vi "Set Socket.vi"(8 "error in (no error)":errorcluster, 11 "Channel Pub in":refnum<class "Channel Pub.lvclass">) -> (0 "error out":errorcluster, 3 "Channel Pub out":refnum<class "Channel Pub.lvclass">)   [LabVIEW 2018, in "Channel Pub.lvclass"]
uses:
  Channel Pub.lvclass
  Communication Channel/Communication Channel Folder/Communication Channel.lvclass
  Socket2/Socket2/Socket2.lvclass
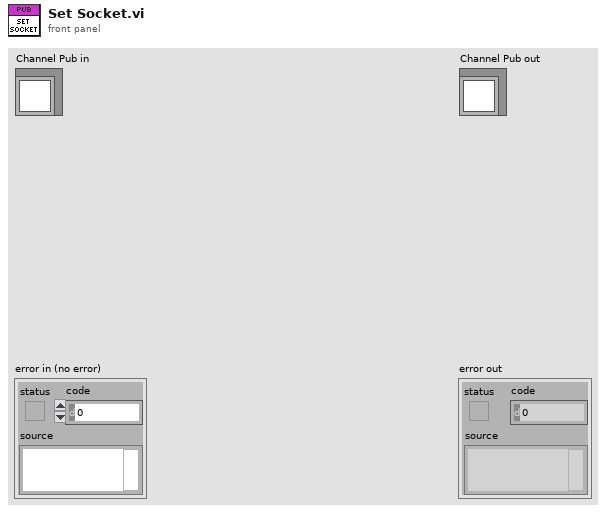
[diagram p1: front panel]
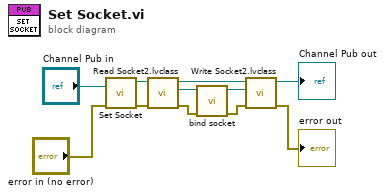
[diagram p0: block diagram]
diagram:
  n1 = call-parent "Set Socket.vi"("error in (no error)"="error in (no error)", "Communication Channel in"="Channel Pub in") -> ("error out"=w3:errorcluster, "Communication Channel out"=w4:refnum<class "Channel Pub.lvclass">)  [unwired: 8 in]
  n2 = call-dynamic "Read Socket2.lvclass.vi"("error in (no error)"=w3, "Communication Channel in"=w4) -> ("error out"=w6:errorcluster, "Socket2.lvclass"=w9:refnum<class "Socket2.lvclass">, "Communication Channel out"=w7:refnum<class "Channel Pub.lvclass">)  [unwired: 7 in]
  n3 = call "bind socket.vi"("error in (no error)"=w6, "Socket in"=w9) -> ("error out"=w5:errorcluster, "Socket out"=w8:refnum<class "Socket2.lvclass">)  [unwired: 8 in]
  n4 = call-dynamic "Write Socket2.lvclass.vi"("error in (no error)"=w5, "Socket2.lvclass"=w8, "Communication Channel in"=w7) -> ("error out"=→"error out":errorcluster, "Communication Channel out"=→"Channel Pub out":refnum<class "Channel Pub.lvclass">)  [unwired: 7 in]
